vi "File Write Size Test.vi"() -> ()   [LabVIEW 2025]
doc: "Author: Scott Hannahs <sth@magnet.fsu.edu>\n\nThis software is licensed for use under the “MIT License\"\nCopyright (c) 2025 Scott Hannahs, sth@sth@magnet.sthnet.net\n\nPermission is hereby granted, free of charge, to any person obtaining a copy of this software and associated documentation files (the \"Software\"), to deal in the Software without restriction, including without limitation the rights to use, copy, modify, merge, publish, distribute, sublicense, and/or sell copies of the Software, and to permit persons to whom the Software is furnished to do so, subject to the following conditions: The above copyright notice and this permission notice shall be included in all copies or substantial portions of the Software.\n\nTHE SOFTWARE IS PROVIDED \"AS IS\", WITHOUT WARRANTY OF ANY KIND, EXPRESS OR IMPLIED, INCLUDING BUT NOT LIMITED TO THE WARRANTIES OF MERCHANTABILITY, FITNESS FOR A PARTICULAR PURPOSE AND NONINFRINGEMENT. IN NO EVENT SHALL THE AUTHORS OR COPYRIGHT HOLDERS BE LIABLE FOR ANY CLAIM, DAMAGES OR OTHER LIABILITY, WHETHER IN AN ACTION OF CONTRACT, TORT OR OTHERWISE, ARISING FROM, OUT OF OR IN CONNECTION WITH THE SOFTWARE OR THE USE OR OTHER DEALINGS IN THE SOFTWARE."
uses:
  Sub Controls/Instrument Properties.ctl
  Sub Controls/Public.ctl
  Sub Controls/Private.ctl
  Sub Controls/Instrument Ref.ctl
  Sub Controls/SystemCheckBox-resize.ctl
panel:
  in  "Column #":i32=10
  out "Array":errorcluster[](array[cluster])
  in  "Data Size (Rows)":i32=100000
  in  "Step Size":i32
  in  "# steps":i32
  out "XY Graph":cluster{dbl[], dbl[]}(graph)
  in  "file path (use dialog)":path=path "/Cell04DataMac/private/tmp/LabVIEW_File_Test.txt"
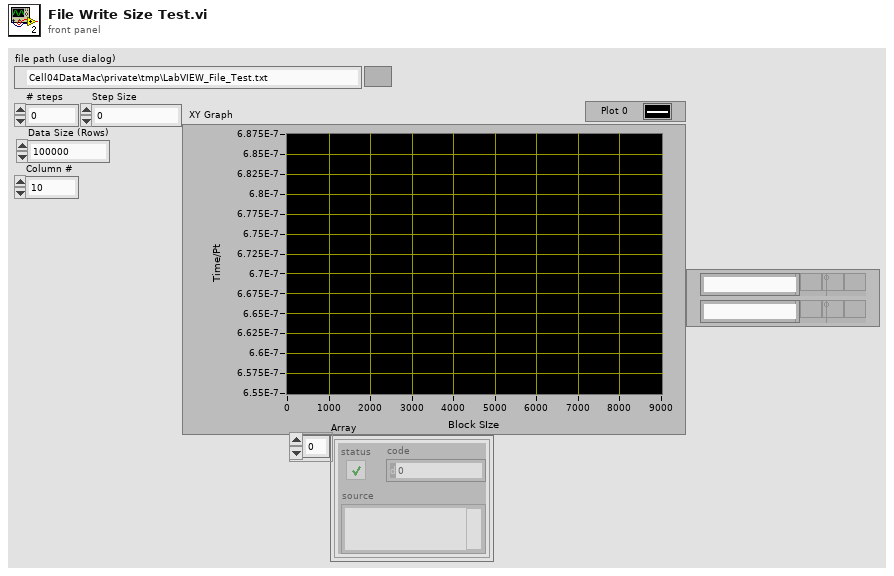
[diagram p1: front panel]
types:
  T1 = enum16{"open", "replace", "create", "open or create", "replace or create", "replace or create with confirmation"}
  T2 = typedef "Instrument Properties.ctl" = cluster{"Public":T3, "Private":T4}
  T3 = typedef "Public.ctl" = cluster{"Column Name":string[], "Trace Color":u32[]}
  T4 = typedef "Private.ctl" = cluster{"Path":path, "VI Refnum":T5, "Name":string, "# of Values":i32, "Scale Factors":dbl[], "Display":T6[], "Offset":dbl[]}
  T5 = typedef "Instrument Ref.ctl" = refnum<vi>
  T6 = typedef "SystemCheckBox-resize.ctl" = bool
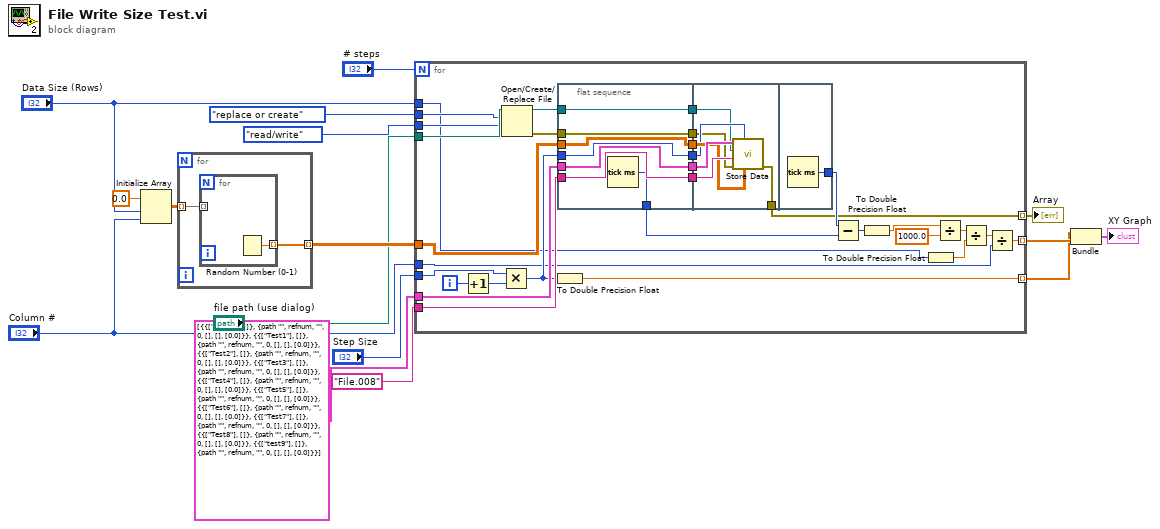
[diagram p0: block diagram]
diagram:
  n1 = Initialize Array(0.0 ("element"), "Data Size (Rows)", "Column #") -> (w13:dbl[][])
  n2 = for {
    tunnel: w13 -> [w18] mode=indexing
    tunnel: [w17] -> w12 mode=indexing
    n3 = for {
      tunnel: w18 -> [_] mode=indexing
      tunnel: [w19] -> w17 mode=indexing
      n4 = Random Number (0-1)() -> (number: 0 to 1=w19:dbl)
    }
  }
  n5 = for {
    N: "# steps" -> [_]
    tunnel: T2[] [{"Public"={"Column Name"=["Test0"], "Trace Color"=[]}, "Private"={"Path"=path "", "VI Refnum"=refnum, "Name"="", "# of Values"=0, "Scale Factors"=[], "Display"=[], "Offset"=[0.0]}}, {"Public"={"Column Name"=["Test1"], "Trace Color"=[]}, "Private"={"Path"=path "", "VI Refnum"=refnum, "Name"="", "# of Values"=0, "Scale Factors"=[], "Display"=[], "Offset"=[0.0]}}, {"Public"={"Column Name"=["Test2"], "Trace Color"=[]}, "Private"={"Path"=path "", "VI Refnum"=refnum, "Name"="", "# of Values"=0, "Scale Factors"=[], "Display"=[], "Offset"=[0.0]}}, {"Public"={"Column Name"=["Test3"], "Trace Color"=[]}, "Private"={"Path"=path "", "VI Refnum"=refnum, "Name"="", "# of Values"=0, "Scale Factors"=[], "Display"=[], "Offset"=[0.0]}}, {"Public"={"Column Name"=["Test4"], "Trace Color"=[]}, "Private"={"Path"=path "", "VI Refnum"=refnum, "Name"="", "# of Values"=0, "Scale Factors"=[], "Display"=[], "Offset"=[0.0]}}, {"Public"={"Column Name"=["Test5"], "Trace Color"=[]}, "Private"={"Path"=path "", "VI Refnum"=refnum, "Name"="", "# of Values"=0, "Scale Factors"=[], "Display"=[], "Offset"=[0.0]}}, {"Public"={"Column Name"=["Test6"], "Trace Color"=[]}, "Private"={"Path"=path "", "VI Refnum"=refnum, "Name"="", "# of Values"=0, "Scale Factors"=[], "Display"=[], "Offset"=[0.0]}}, {"Public"={"Column Name"=["Test7"], "Trace Color"=[]}, "Private"={"Path"=path "", "VI Refnum"=refnum, "Name"="", "# of Values"=0, "Scale Factors"=[], "Display"=[], "Offset"=[0.0]}}, {"Public"={"Column Name"=["Test8"], "Trace Color"=[]}, "Private"={"Path"=path "", "VI Refnum"=refnum, "Name"="", "# of Values"=0, "Scale Factors"=[], "Display"=[], "Offset"=[0.0]}}, {"Public"={"Column Name"=["test9"], "Trace Color"=[]}, "Private"={"Path"=path "", "VI Refnum"=refnum, "Name"="", "# of Values"=0, "Scale Factors"=[], "Display"=[], "Offset"=[0.0]}}] ("Instrument List In") -> [w47]
    tunnel: "File.008" ("File Name") -> [w46]
    tunnel: w12 -> [w45]
    tunnel: [w21] -> w10 mode=indexing
    tunnel: "Step Size" -> [w42]
    tunnel: [w25] -> w7 mode=indexing
    tunnel: "file path (use dialog)" -> [w33]
    tunnel: T1."replace or create" ("operation (0:open)") -> [w32]
    tunnel: enum16{"read/write", "read-only", "write-only"}."read/write" ("access (0:read/write)") -> [w31]
    tunnel: "Data Size (Rows)" -> [w29]
    tunnel: [w38] -> w2 mode=indexing
    tunnel: "Column #" -> [w20]
    i -> [w41]
    n6 = Increment(x=w41) -> (x+1=w40:i32)
    n7 = Multiply(x=w42, y=w40) -> (x*y=w37:i32)
    n8 = Open/Create/Replace File(file path (use dialog)=w33, operation (0:open)=w32, access (0:read/write)=w31) -> (refnum out=w22:refnum<file>, error out=w34:errorcluster)  [unwired: 3 in, 1 out]
    n9 = To Double Precision Float(number=w37) -> (double precision float=w25:dbl)
    n10 = flat-sequence {
      tunnel: w45 -> [w55]
      tunnel: w46 -> [w56]
      tunnel: w47 -> [w57]
      tunnel: [w57] -> w50
      tunnel: [w56] -> w49
      tunnel: [w55] -> w48
      tunnel: [w54] -> w43
      tunnel: w37 -> [w53]
      tunnel: [w53] -> w36
      tunnel: w34 -> [w52]
      tunnel: [w52] -> w35
      tunnel: [w51] -> w23
      tunnel: w22 -> [w51]
      tunnel: w50 -> [w64]
      tunnel: w49 -> [w63]
      tunnel: w48 -> [w62]
      tunnel: [w61] -> w38
      tunnel: w36 -> [w60]
      tunnel: w35 -> [w59]
      tunnel: w23 -> [w58]
      tunnel: [w65] -> w44
      frame #0 {
        n11 = Tick Count (ms)() -> (millisecond timer value=w54:u32)
      }
      frame #1 {
        n12 = call "Store Data.vi"("All Data"=w62, "Block Size"=w60, "error in"=w59, "File Name"=w63, "Byte Stream File in"=w58, "Instrument List In"=w64) -> ("error out"=w61:errorcluster)  [unwired: 4 in, 1 out]
      }
      frame #2 {
        n13 = Tick Count (ms)() -> (millisecond timer value=w65:u32)
      }
    }
    n14 = Subtract(x=w44, y=w43) -> (x-y=w39:u32)
    n15 = To Double Precision Float(number=w39) -> (double precision float=w24:dbl)
    n16 = To Double Precision Float(number=w29) -> (double precision float=w26:dbl)
    n17 = Divide(x=w24, y=1000.0) -> (x/y=w28:dbl)
    n18 = Divide(x=w28, y=w26) -> (x/y=w30:dbl)
    n19 = Divide(x=w30, y=w20) -> (x/y=w21:dbl)
  }
  "Array" <- w2
  n20 = Bundle(w7, w10) -> (→"XY Graph":cluster{dbl[], dbl[]})  [unwired: 1 in]
